vi "Run.vi"(8 "error in":errorcluster, 10 "Execution Plan":T1={"Exe Path"=path "", "Args"=[], "Timeout"=-1}, 11 "Process Executor Mock in":refnum<class "Process Executor Mock.lvclass">) -> (0 "error out":errorcluster, 3 "Process Executor Mock out":refnum<class "Process Executor Mock.lvclass">)   [LabVIEW 2025, in "Process Executor Mock.lvclass"]
doc: "Mocks the Process Executor for testing purposes. In normal execution this VI does not produce an error. If an error is provided as input, it is passed on."
uses:
  Process Executor Mock.lvclass
  Type Definitions/Execution Plan--cluster.ctl
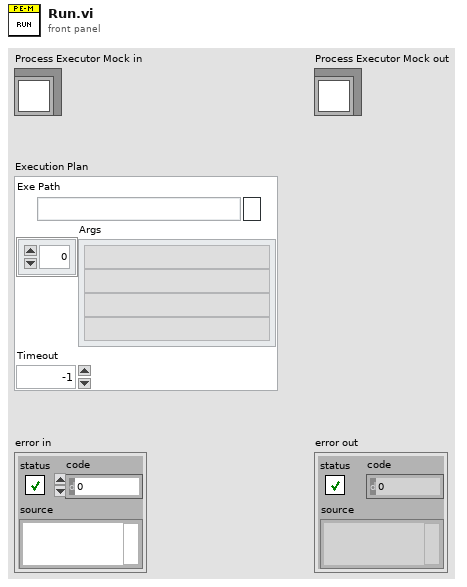
[diagram p1: front panel]
types:
  T1 = typedef "Execution Plan--cluster.ctl" = cluster{"Exe Path":path, "Args":string[], "Timeout":i32}
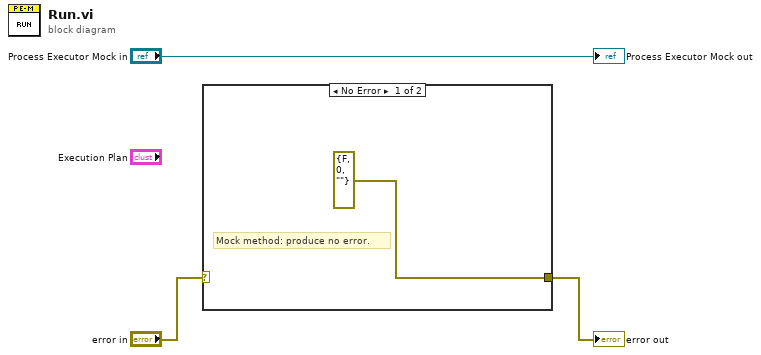
[diagram p0: block diagram]
diagram:
  n1 = case shown="No Error" "error in" {
    selector: "error in" -> [_ w5]
    tunnel: [errorcluster {"status"=FALSE, "code"=0, "source"=""} ("error out") w5] -> w2
    frame No Error {
      # "Mock method: produce no error."
    }
    frame Error {
      # "Pass error unchanged"
    }
  }
  "error out" <- w2
  "Process Executor Mock out" <- "Process Executor Mock in"
